vi "Print.vi"(11 "CANopen Message in":refnum<class "CANopen Message.lvclass">) -> (2 "Message":string, 3 "CANopen Message out":refnum<class "CANopen Message.lvclass">)   [LabVIEW 2024, in "CANopen Master.lvlib" / "CANopen Message.lvclass"]
uses:
  CANopen Message.lvclass
  CANopen Message.lvclass/CANopen Message.ctl
  <vilib>/Utility/error.llb/whitespace.ctl
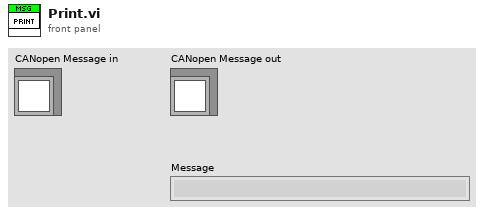
[diagram p1: front panel]
types:
  T1 = typedef "whitespace.ctl" = u16
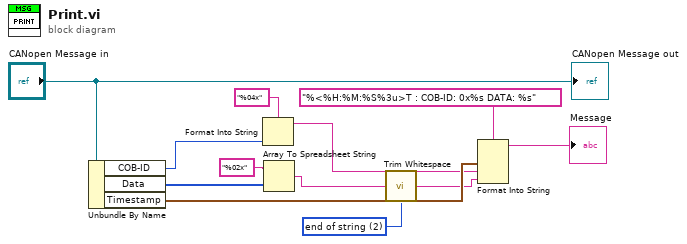
[diagram p0: block diagram]
diagram:
  w2 = T1 2 items=["both", "start of string", "end of string"] ("location (both)")
  n1 = Unbundle By Name("CANopen Message in") -> ("COB-ID"=w8:u32, "Data"=w9:u8[], "Timestamp"=w11:timestamp)
  n2 = Format Into String(format string="%04x", w8) -> (resulting string=w7:string)  [unwired: 2 in, 1 out]
  n3 = Array To Spreadsheet String(array=w9, 3:"%02x" ("format string")) -> (spreadsheet string=w4:string)  [unwired: 1 in]
  n4 = call <vilib>:"Trim Whitespace.vi"("string"=w4, "location (both)"=w2) -> ("trimmed string"=w3:string)
  n5 = Format Into String(format string="%<%H:%M:%S%3u>T : COB-ID: 0x%s DATA: %s", w11, w7, w3) -> (resulting string=→"Message":string)  [unwired: 2 in, 1 out]
  "CANopen Message out" <- "CANopen Message in"
